vi "ACT_Loop.vi"() -> ()   [LabVIEW 2023, in "Shooter FX_ACT.lvlib"]
uses:
  Shooter FX_ACT.lvlib
  RoboRIO Utilities/Global_STOP.vi
  ENUM_ACT_Action.ctl
  ENUM_ACT_State.ctl
  Global_CMD_ACT_Data In.vi
  Global_ACT_Data Out.vi
  Cluster_CMD_ACT_Data.ctl
  <vilib>/Rock Robotics/WPI/MotorControl/WPI_MotorControlType.ctl
  <vilib>/Rock Robotics/SystemInterfaces/DIO/FPGA_DIOPWMChannel.ctl
  <vilib>/Rock Robotics/WPI/PWM/WPI_PWMDeadband.ctl
  <vilib>/Rock Robotics/SystemInterfaces/DIO/FPGA_DIOChannel.ctl
  <vilib>/Rock Robotics/WPI/MotorControl/WPI_MotorControlDeviceRef.ctl
  Shared Code/TypeDefs/Cluser_CAN Data.ctl
  <vilib>/Rock Robotics/WPI/ThirdParty/Phoenix-LabVIEW/Motor Controller/Controls/CTRE_Phoenix_MotorControl_NeutralMode.ctl
  Shared Code/TypeDefs/Cluster_FWD  REV Values.ctl
  Shared Code/TypeDefs/Cluster_PID Gains.ctl
  Cluster_Config HW Values.ctl
  b5508d6c-c1cc-4273-80c5-2077d34e1483.vi
  5f725c2a-0ce1-4524-8967-e83b15fdce90.vi
  <vilib>/Rock Robotics/WPI/ThirdParty/Phoenix-LabVIEW/Motor Controller/Controls/CTRE_Phoenix_MotorControl_ControlMode.ctl
  Shared Code/TypeDefs/Cluster_FX CloseLoop Values.ctl
  Shared Code/TypeDefs/Cluster_FX Current Values.ctl
  Cluster_HW Output Values.ctl
  ENUM_CMD_Mode Select.ctl
  Shared Code/TypeDefs/Cluster_FX Sensor Values.ctl
  4f1f8321-3dc8-4b28-8619-20673fc77ec2.vi
  Cluster_SW Output Data.ctl
  Cluster_Config SW Values.ctl
  36677ea0-a1a5-47a3-bc56-4475cb7c281e.vi
  573e44c0-11f4-4bd9-ad56-904ec25dba75.vi
  e7494af9-f670-4352-9dfa-ae6ce50709ea.vi
  6201c2b1-dcd8-4430-86f1-9b4ee56c7753.vi
  Shared Code/TypeDefs/Cluser_FX Config_Current Limits.ctl
  Shared Code/TypeDefs/Cluster_FX SLOT PID Config.ctl
  <vilib>/Rock Robotics/WPI/ThirdParty/Phoenix-LabVIEW/Motor Controller/Controls/CTRE_Phoenix_MotorControl_TalonFXInvertType.ctl
  Shared Code/TypeDefs/Cluster_Config FX Motor Output.ctl
  Shared Code/TypeDefs/Cluster_FX Voltage Values.ctl
  2024 Intake/Global_CMD_ACT_Data In.vi
  2024 Intake/Intake_ACT.lvlib
  2024 Intake/ENUM_Shooter_Mode.ctl
  2024 Intake/Cluster_CMD_ACT_Data.ctl
panel:
  in  "Enable 1":bool
  out "STATE":T1
  in  "CMD Override":T2(tab)
  in  "Percent Out":dbl(slide) scale=-1.0..1.0
  in  "Position Counts":dbl
  in  "Velocity Value":dbl
  out "Current Time":timestamp
  in  "SW Config":T3={"Ver"=0, "Shooting Speed (RPM)"=1000.0}
  out "SW Output":T4
  out "Sensor Read time":dbl format="%.3g"
  out "HW Sensors":T5
  in  "Read Saved Config":bool
  in  "Update Config":bool
  in  "HW Config":T10 {"CL"."Gains"."F" format="%#.8f"; "CL"."Gains"."D" format="%#.8f"; "CL"."Gains"."I" format="%#.8f"; "CL"."Gains"."P" format="%#.8f"; "Output"."Min"."REV" format="%.2f"; "Output"."Min"."FWD" format="%.2f"; "Output"."Max"."REV" format="%.2f"; "Output"."Max"."FWD" format="%.2f"}
  out "CMD":T19
  out "Cycle Time (S)":dbl format="%.3g"
  # "Teleop - Auto"
  # "Shoot at Target Speed"
  # "STOP"
  # "Tune Output\nto 1023 Max"
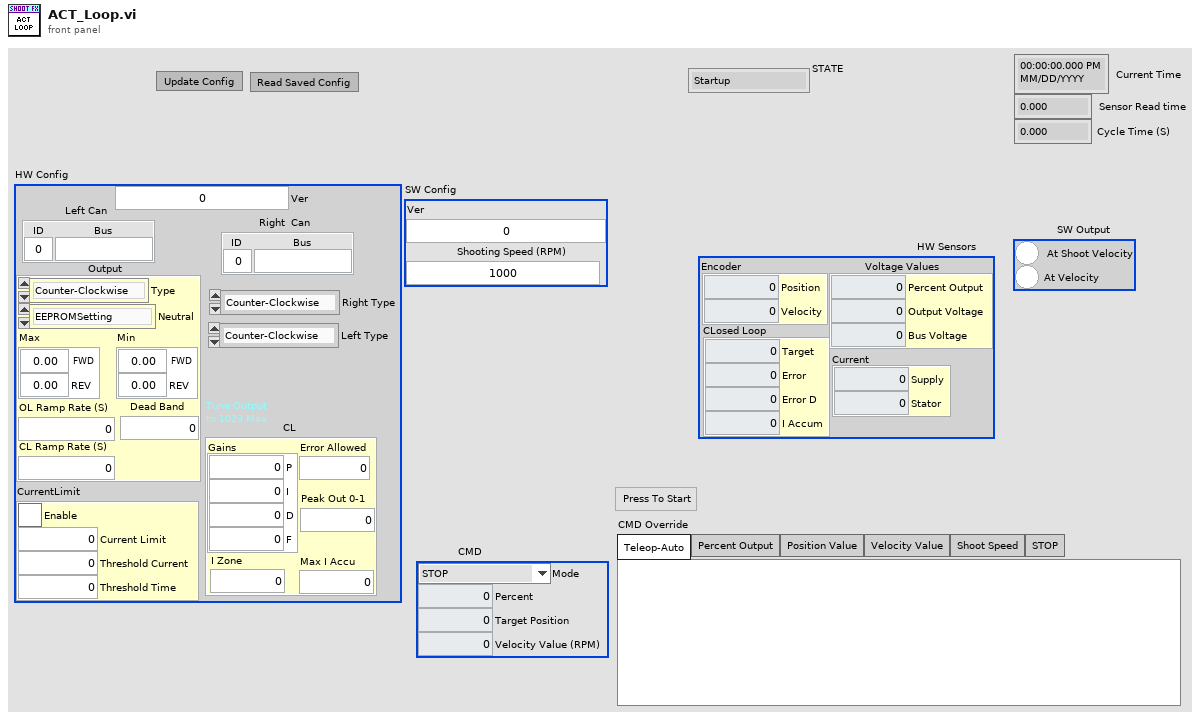
[diagram p1: front panel]
types:
  T1 = typedef "Shooter FX_ACT.lvlib/ENUM_ACT_State.ctl" = enum16{"Startup", "Configuring", "Stopping", "Moving Percent Out", "Moving to Position", "Shutdown", "Moving Velocity", "Moving to Shoot Vel", "Shooting"}
  T2 = enum32{"Teleop-Auto", "Percent Output", "Position Value", "Velocity Value", "Shoot Speed", "STOP"}
  T3 = typedef "Shooter FX_ACT.lvlib/Cluster_Config SW Values.ctl" = cluster{"Ver":u64, "Shooting Speed (RPM)":dbl}
  T4 = typedef "Shooter FX_ACT.lvlib/Cluster_SW Output Data.ctl" = cluster{"At Shoot Velocity":bool, "At Velocity":bool}
  T5 = typedef "Shooter FX_ACT.lvlib/Cluster_HW Output Values.ctl" = cluster{"Encoder":T6, "Current":T7, "CLosed Loop":T8, "Voltage Values":T9}
  T6 = typedef "Cluster_FX Sensor Values.ctl" = cluster{"Position":i32, "Velocity":i32}
  T7 = typedef "Cluster_FX Current Values.ctl" = cluster{"Supply":dbl, "Stator":dbl}
  T8 = typedef "Cluster_FX CloseLoop Values.ctl" = cluster{"Target":dbl, "Error":i32, "Error D":dbl, "I Accum":dbl}
  T9 = typedef "Cluster_FX Voltage Values.ctl" = cluster{"Percent Output":dbl, "Output Voltage":dbl, "Bus Voltage":dbl}
  T10 = typedef "Shooter FX_ACT.lvlib/Cluster_Config HW Values.ctl" = cluster{"Ver":u64, "Right  Can":T11, "Output":T12, "CL":T16, "CurrentLimit":T18, "Left Can":T11, "Right Type":T13, "Left Type":T13}
  T11 = typedef "Cluser_CAN Data.ctl" = cluster{"ID":u8, "Bus":string}
  T12 = typedef "Cluster_Config FX Motor Output.ctl" = cluster{"Type":T13, "Neutral":T14, "Max":T15, "Min":T15, "OL Ramp Rate (S)":dbl, "Dead Band":dbl, "CL Ramp Rate (S)":dbl}
  T13 = typedef "CTRE_Phoenix_MotorControl_TalonFXInvertType.ctl" = enum16{"Counter-Clockwise", "Clockwise"}
  T14 = typedef "CTRE_Phoenix_MotorControl_NeutralMode.ctl" = enum8{"EEPROMSetting", "Override to Coast", "Override to Brake"}
  T15 = typedef "Cluster_FWD  REV Values.ctl" = cluster{"FWD":dbl, "REV":dbl}
  T16 = typedef "Cluster_FX SLOT PID Config.ctl" = cluster{"Gains":T17, "Error Allowed":dbl, "I Zone":dbl, "Peak Out 0-1":dbl, "Max I Accu":dbl}
  T17 = typedef "Cluster_PID Gains.ctl" = cluster{"P":dbl, "I":dbl, "D":dbl, "F":dbl}
  T18 = typedef "Cluser_FX Config_Current Limits.ctl" = cluster{"Enable":bool, "Current Limit":dbl, "Threshold Current":dbl, "Threshold Time":dbl}
  T19 = typedef "Shooter FX_ACT.lvlib/Cluster_CMD_ACT_Data.ctl" = cluster{"Mode":T20, "Percent":dbl, "Target Position":dbl, "Velocity Value (RPM)":dbl}
  T20 = typedef "Shooter FX_ACT.lvlib/ENUM_CMD_Mode Select.ctl" = enum16{"STOP", "PercentOut", "Positon Value", "Velocity Value", "Shoot Speed", "Auto Shoot"}
  T21 = typedef "WPI_MotorControlDeviceRef.ctl" = cluster{"DeviceStatus":errorcluster, "Type":T22, "PWM":cluster{"PWM Channel":T23, "DeadBand":T24}, "CAN":cluster{"Device Number":u8, "SetOutput VI Ref":variant, "GetOutput VI Ref":variant, "Enable VI Ref":variant, "Disable VI Ref":variant, "Data":variant}, "Invert":bool, "DIO PWM":cluster{"PWM \"Enable\" Channel":T23, "DIOChannel":T25, "PWM Rate":dbl}}
  T22 = typedef "WPI_MotorControlType.ctl" = enum16{"PWM", "CAN", "DIO PWM"}
  T23 = typedef "FPGA_DIOPWMChannel.ctl" = enum8{"PWM 0", "PWM 1", "PWM 2", "PWM 3", "PWM 4", "PWM 5", "PWM 6", "PWM 7", "PWM 8", "PWM 9", "PWM MXP 0", "PWM MXP 1", "PWM MXP 2", "PWM MXP 3", "PWM MXP 4", "PWM MXP 5", "PWM MXP 6", "PWM MXP 7", "PWM MXP 8", "PWM MXP 9", "Invalid"}
  T24 = typedef "WPI_PWMDeadband.ctl" = cluster{"Name":string, "maxPositivePwm":i32, "minPositivePwm":i32, "centerPwm":i32, "maxNegativePwm":i32, "minNegativePwm":i32, "angularRange":u16}
  T25 = typedef "FPGA_DIOChannel.ctl" = enum8{"DIO 0", "DIO 1", "DIO 2", "DIO 3", "DIO 4", "DIO 5", "DIO 6", "DIO 7", "DIO 8", "DIO 9", "DIO MXP 0", "DIO MXP 1", "DIO MXP 2", "DIO MXP 3", "DIO MXP 4", "DIO MXP 5", "DIO MXP 6", "DIO MXP 7", "DIO MXP 8", "DIO MXP 9", "DIO MXP 10", "DIO MXP 11", "DIO MXP 12", "DIO MXP 13", "DIO MXP 14", "DIO MXP 15", "SPI Port CS1", "SPI Port CS2", "SPI Port CS3", "SPI Port MISO", "SPI Port MOSI", "Invalid"}
  T26 = typedef "Intake_ACT.lvlib/Cluster_CMD_ACT_Data.ctl" = cluster{"Mode":T27, "Speed Value":dbl}
  T27 = typedef "Intake_ACT.lvlib/ENUM_Shooter_Mode.ctl" = enum16{"Stop", "Speed Percent", "Speed RPM"}
  T28 = typedef "CTRE_Phoenix_MotorControl_ControlMode.ctl" = u16
  T29 = cluster{"Team Files Folder":path, "Left Motor":T21, "Right Motor Ref":T21, "State":T1, "Previous State":T1, "Current Time":timestamp, "Previous Time":timestamp, "Start Time":timestamp, "Target Time (ms)":u32, "Cycle Time(S)":dbl, "Update Display":bool, "ACT Input":T19, "HW Config":T10, "SW Config":T3, "Max # Of Config Tries":i32, "HW Out":T5, "SW Out":T4, "CAN Timeout":u32, "FX Mode":T28, "FX Set Value":dbl, "CMDIntake":T26}
  T30 = typedef "Shooter FX_ACT.lvlib/ENUM_ACT_Action.ctl" = enum16{"No Action", "Reset Time", "Reset All", "Config HW File Read", "Config HW File Save", "Config SW File Read", "Config SW File Save", "Config From FP", "Config HW Get", "Config HW Set", "Open HW Only", "Control FX Stop", "Control FX Set Percent Out", "Control FX Set Pos Value", "Control FX Set Velocity Value", "Control FX Set STOP", "Encoder Set to Zero", "Set Shooter Velocity"}
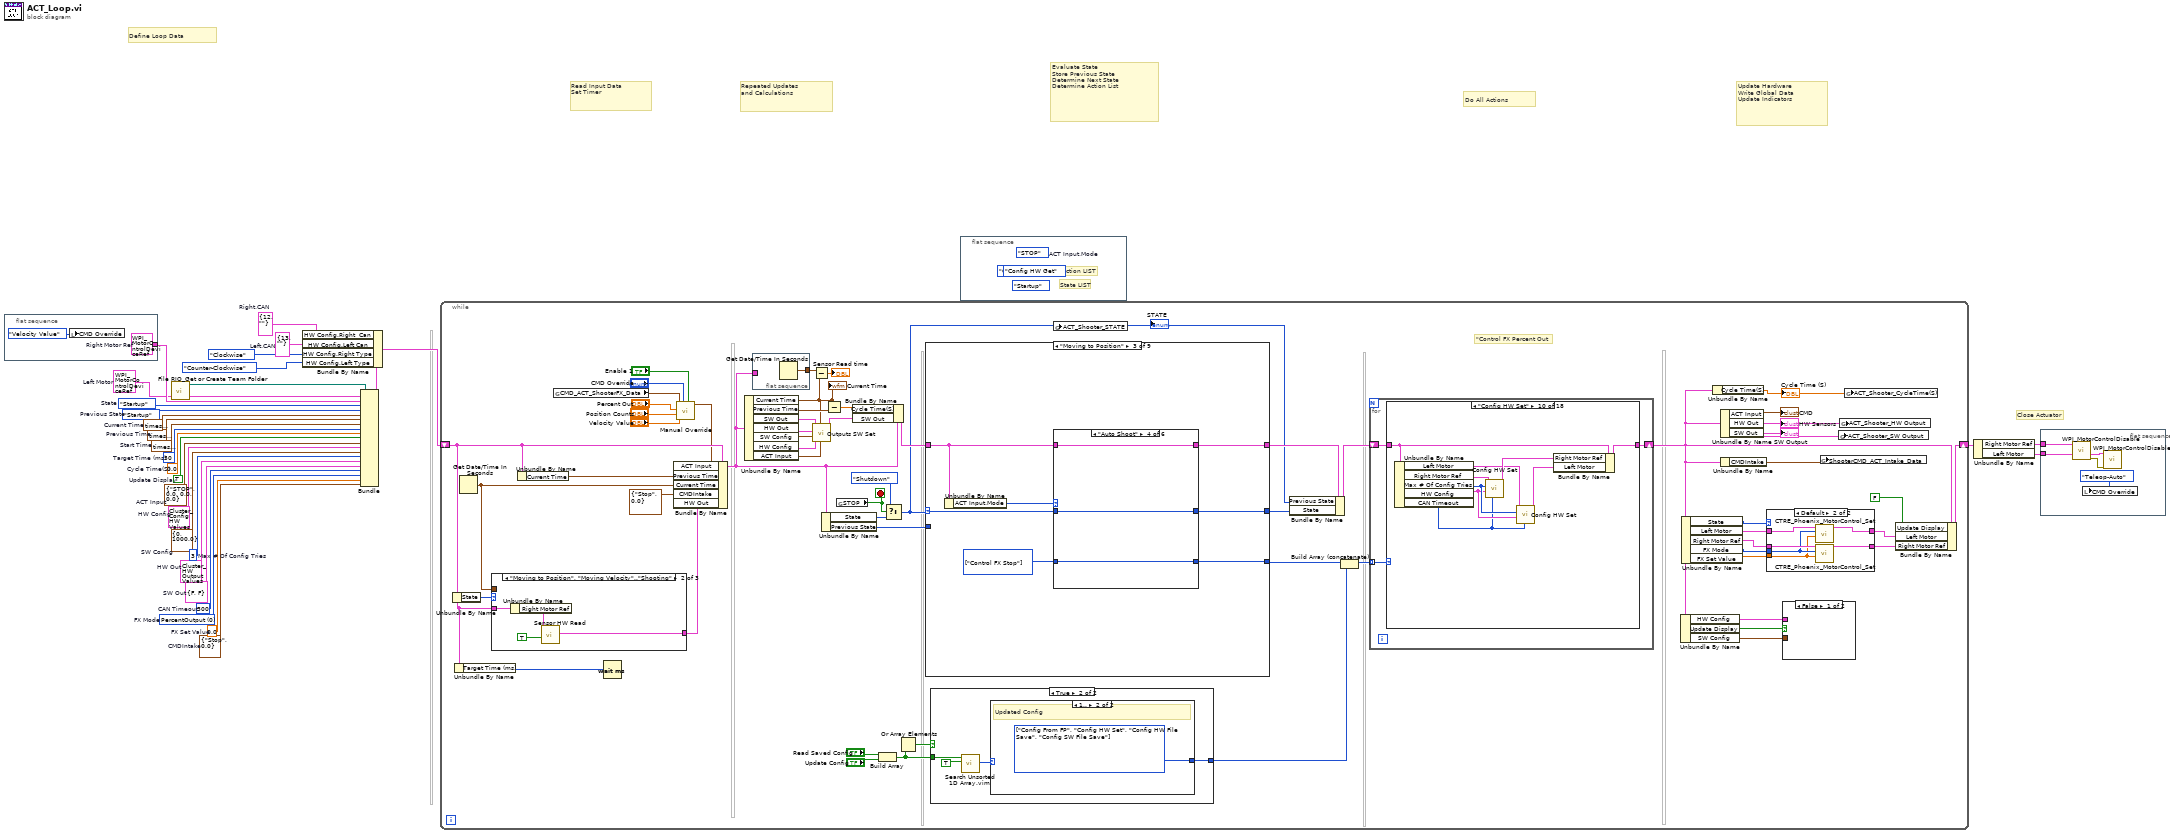
[diagram p0: block diagram]
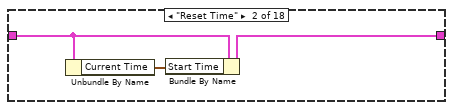
[diagram p3: hidden frame]
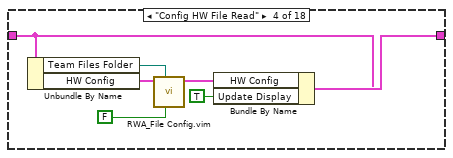
[diagram p5: hidden frame]
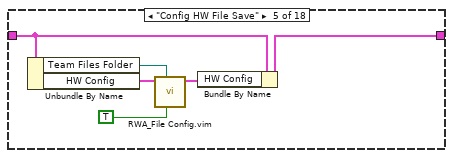
[diagram p6: hidden frame]
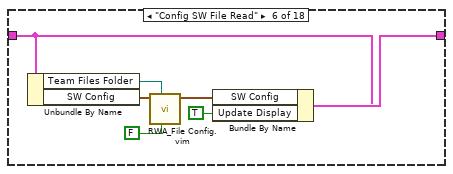
[diagram p7: hidden frame]
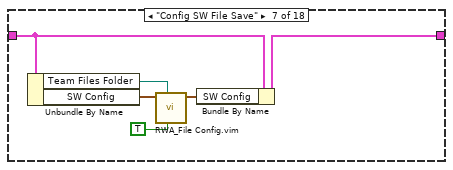
[diagram p8: hidden frame]
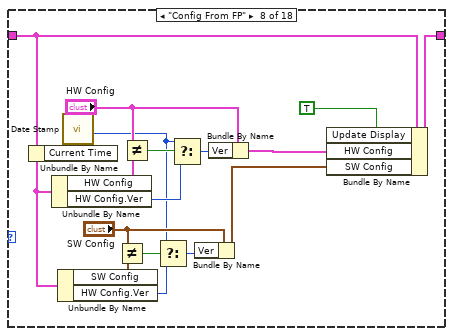
[diagram p9: hidden frame]
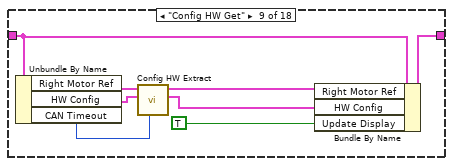
[diagram p10: hidden frame]
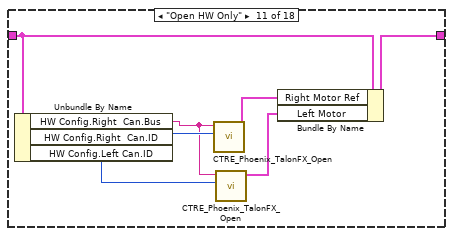
[diagram p11: hidden frame]
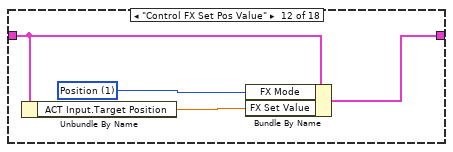
[diagram p12: hidden frame]
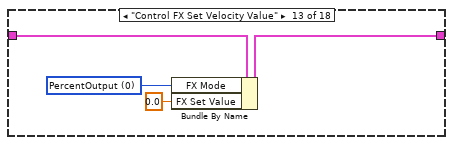
[diagram p13: hidden frame]
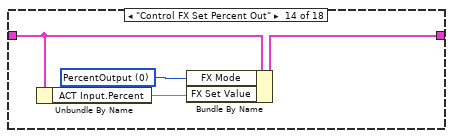
[diagram p14: hidden frame]
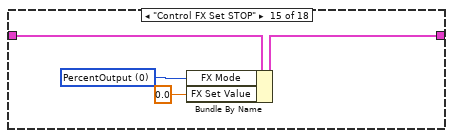
[diagram p15: hidden frame]
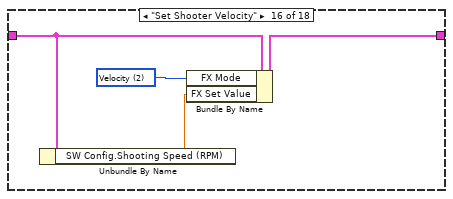
[diagram p16: hidden frame]
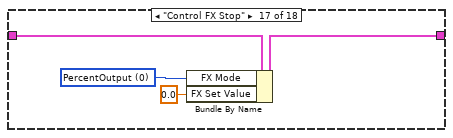
[diagram p17: hidden frame]
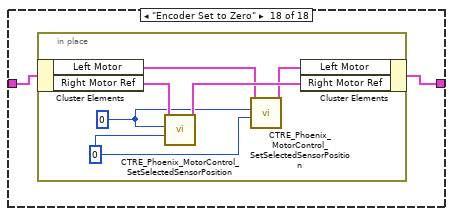
[diagram p18: hidden frame]
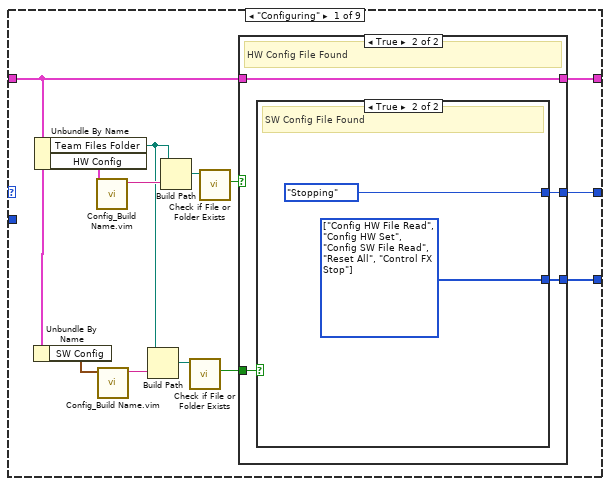
[diagram p19: hidden frame]
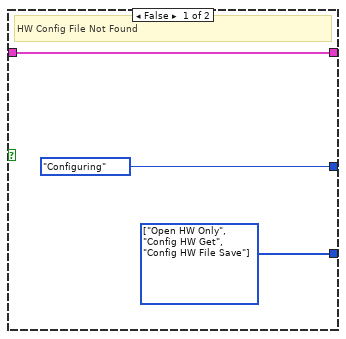
[diagram p20: hidden frame]
diagram:
  w3 = T11 {"ID"=13, "Bus"=""}  # Left.CAN
  w5 = T21 {"DeviceStatus"={"status"=FALSE, "code"=0, "source"=""}, "Type"=enum."PWM", "PWM"={"PWM Channel"=enum."PWM 1", "DeadBand"={"Name"="", "maxPositivePwm"=0, "minPositivePwm"=0, "centerPwm"=0, "maxNegativePwm"=0, "minNegativePwm"=0, "angularRange"=0}}, "CAN"={"Device Number"=0, "SetOutput VI Ref"=variant(enum8{"Percent VBus", "Current", "Speed", "Position", "Voltage"} enum."Percent VBus"), "GetOutput VI Ref"=variant(refnum<k1> refnum), "Enable VI Ref"=variant(dbl 12.0), "Disable VI Ref"=variant(enum8{"Percent VBus", "Speed", "Position", "Slave", "Unchanged / Invalid", "Voltage Compensation", "Current", "Motion Profile"} enum."Percent VBus"), "Data"=variant}, "Invert"=FALSE, "DIO PWM"={"PWM \"Enable\" Channel"=enum."Invalid", "DIOChannel"=enum."Invalid", "PWM Rate"=0.0}}  # Left Motor
  w6 = T26 {"Mode"=enum."Stop", "Speed Value"=0.0}  # CMDIntake
  w7 = T3 {"Ver"=0, "Shooting Speed (RPM)"=1000.0}  # SW Config
  w16 = T10 {"Ver"=0, "Right  Can"={"ID"=0, "Bus"=""}, "Output"={"Type"=enum."Counter-Clockwise", "Neutral"=enum."EEPROMSetting", "Max"={"FWD"=0.0, "REV"=0.0}, "Min"={"FWD"=0.0, "REV"=0.0}, "OL Ramp Rate (S)"=0.0, "Dead Band"=0.0, "CL Ramp Rate (S)"=0.0}, "CL"={"Gains"={"P"=0.0, "I"=0.0, "D"=0.0, "F"=0.0}, "Error Allowed"=0.0, "I Zone"=0.0, "Peak Out 0-1"=0.0, "Max I Accu"=0.0}, "CurrentLimit"={"Enable"=FALSE, "Current Limit"=0.0, "Threshold Current"=0.0, "Threshold Time"=0.0}, "Left Can"={"ID"=0, "Bus"=""}, "Right Type"=enum."Counter-Clockwise", "Left Type"=enum."Counter-Clockwise"}  # HW Config
  w14 = T4 {"At Shoot Velocity"=FALSE, "At Velocity"=FALSE}  # SW Out
  w15 = T5 {"Encoder"={"Position"=0, "Velocity"=0}, "Current"={"Supply"=0.0, "Stator"=0.0}, "CLosed Loop"={"Target"=0.0, "Error"=0, "Error D"=0.0, "I Accum"=0.0}, "Voltage Values"={"Percent Output"=0.0, "Output Voltage"=0.0, "Bus Voltage"=0.0}}  # HW Out
  w10 = 0.0  # FX Set Value
  w11 = T28 0 items=["PercentOutput"=0, "Position"=1, "Velocity"=2, "Current"=3, "Follower"=5, "MotionProfile"=6, "MotionMagic"=7, "MotionProfileArc"=10, "Disabled"=15]  # FX Mode
  w9 = u32 300  # CAN Timeout
  w8 = 3  # Max # Of Config Tries
  w18 = TRUE  # Update Display
  w19 = T11 {"ID"=12, "Bus"=""}  # Right.CAN
  w24 = 0.0  # Cycle Time(S)
  w25 = ENUM_ACT_State."Startup"  # Previous State
  w26 = timestamp(0 s since 1904-01-01)  # Previous Time
  w27 = u32 50  # Target Time (ms)
  w13 = T19 {"Mode"=enum."STOP", "Percent"=0.0, "Target Position"=0.0, "Velocity Value (RPM)"=0.0}  # ACT Input
  w28 = timestamp(0 s since 1904-01-01)  # Start Time
  w29 = timestamp(0 s since 1904-01-01)  # Current Time
  w30 = ENUM_ACT_State."Startup"  # State
  # "Close Actuator"
  # "Define Loop Data"
  # "Repeated Updates\nand Calculations"
  # "Read Input Data\nSet Timer"
  # "Evaluate State\nStore Previous State\nDetermine Next State\nDetermine Action List"
  # "Do All Actions"
  # "Update Hardware\nWrite Global Data\nUpdate Indicators"
  n1 = flat-sequence {
    tunnel: [w32] -> w20
    frame #0 {
      w32 = T21 {"DeviceStatus"={"status"=FALSE, "code"=0, "source"=""}, "Type"=enum."PWM", "PWM"={"PWM Channel"=enum."PWM 1", "DeadBand"={"Name"="", "maxPositivePwm"=0, "minPositivePwm"=0, "centerPwm"=0, "maxNegativePwm"=0, "minNegativePwm"=0, "angularRange"=0}}, "CAN"={"Device Number"=0, "SetOutput VI Ref"=variant(enum8{"Percent VBus", "Current", "Speed", "Position", "Voltage"} enum."Percent VBus"), "GetOutput VI Ref"=variant(refnum<k1> refnum), "Enable VI Ref"=variant(dbl 12.0), "Disable VI Ref"=variant(enum8{"Percent VBus", "Speed", "Position", "Slave", "Unchanged / Invalid", "Voltage Compensation", "Current", "Motion Profile"} enum."Percent VBus"), "Data"=variant}, "Invert"=FALSE, "DIO PWM"={"PWM \"Enable\" Channel"=enum."Invalid", "DIOChannel"=enum."Invalid", "PWM Rate"=0.0}}  # Right Motor Ref
      n2 = local write "CMD Override"(T2."Velocity Value" ("CMD Override")) -> ()
    }
  }
  n3 = call "File RIO_Get or Create Team Folder.vi"() -> ("Team Files Folder"=w12:path)  [unwired: 10 in, 1 out]
  n4 = Bundle("Team Files Folder"=w12, "Left Motor"=w5, "Right Motor Ref"=w20, "State"=w30, "Previous State"=w25, "Current Time"=w29, "Previous Time"=w26, "Start Time"=w28, "Target Time (ms)"=w27, "Cycle Time(S)"=w24, "Update Display"=w18, "ACT Input"=w13, "HW Config"=w16, "SW Config"=w7, "Max # Of Config Tries"=w8, "HW Out"=w15, "SW Out"=w14, "CAN Timeout"=w9, "FX Mode"=w11, "FX Set Value"=w10, "CMDIntake"=w6) -> (w22:T29)  [unwired: 1 in]
  n5 = Bundle By Name(cluster=w22, "HW Config.Right  Can"=w19, "HW Config.Left Can"=w3, "HW Config.Right Type"=CTRE_Phoenix_MotorControl_TalonFXInvertType."Clockwise", "HW Config.Left Type"=CTRE_Phoenix_MotorControl_TalonFXInvertType."Counter-Clockwise") -> (w21:T29)
  n6 = while {
    shift-right: [w76] -> w23
    shift-left: w21 -> [w47]
    stop <- w89 stop-if-true
    # "\"Control FX Percent Out"
    n7 = Unbundle By Name(w47) -> ("State"=w67:T1)
    n8 = Unbundle By Name(w47) -> ("Target Time (ms)"=w86:u32)
    n9 = Get Date/Time In Seconds() -> (seconds since 1Jan1904=w63:timestamp)
    n10 = case shown="\"Moving to Position\", \"Moving Velocity\"..\"Shooting\"" w67 {
      tunnel: w47 -> [w401 w405 _]
      tunnel: w63 -> [_ _ _]
      tunnel: [w398 w402 _] -> w48
      frame "Stopping", "Moving Percent Out" {
        n11 = Unbundle By Name(w401) -> ("Right Motor Ref"=w400:T21)
        n12 = call "Sensor HW Read.vi"("CloseLoop"=FALSE ("Read Closed Loop"), "PhoenixMotorControlDevRef"=w400) -> ("Sensor Values Out"=w398:T5)  [unwired: 7 in, 2 out]
      }
      frame "Moving to Position", "Moving Velocity".."Shooting" {
        n13 = Unbundle By Name(w405) -> ("Right Motor Ref"=w404:T21)
        n14 = call "Sensor HW Read.vi"("CloseLoop"=TRUE ("Read Closed Loop"), "PhoenixMotorControlDevRef"=w404) -> ("Sensor Values Out"=w402:T5)  [unwired: 7 in, 2 out]
      }
      frame "Startup", "Configuring", "Shutdown" {
      }
    }
    n15 = Unbundle By Name(w47) -> ("Current Time"=w85:timestamp)
    n16 = global read "Global_CMD_ACT_Data In.vi" "CMD_ACT_ShooterFX_Data"() -> (w44:T19)
    n17 = Wait (ms)(milliseconds to wait=w86) -> ()  [unwired: 1 out]
    n18 = call "Manual Override.vi"("Enable"="Enable 1", "CMD Override"="CMD Override", "Velocity Data"="Velocity Value", "Position Data"="Position Counts", "Percent Out Data"="Percent Out", "Auto CMD"=w44) -> ("OverRide Command Out"=w46:T19)  [unwired: 5 in]
    n19 = Bundle By Name(cluster=w47, "ACT Input"=w46, "Previous Time"=w85, "Current Time"=w63, "CMDIntake"=T26 {"Mode"=enum."Stop", "Speed Value"=0.0}, "HW Out"=w48) -> (w49:T29)
    n20 = Unbundle By Name(w49) -> ("Current Time"=w53:timestamp, "Previous Time"=w83:timestamp, "SW Out"=w56:T4, "HW Out"=w54:T5, "SW Config"=w52:T3, "HW Config"=w51:T10, "ACT Input"=w41:T19)
    "Current Time" <- w53
    n21 = flat-sequence {
      tunnel: [w93] -> w65
      tunnel: w49 -> [_]
      frame #0 {
        n22 = Get Date/Time In Seconds() -> (seconds since 1Jan1904=w93:timestamp)
      }
    }
    n23 = Subtract(x=w65, y=w53) -> (x-y=→"Sensor Read time":dbl)
    n24 = call "Outputs SW Set.vi"("CMD_ACT_Tempplate Data"=w41, "Current Time"=w53, "HW Config"=w51, "SW Config"=w52, "Sensor Values"=w54, "SW Output"=w56) -> ("SW Output Out"=w55:T4)  [unwired: 5 in]
    n25 = Unbundle By Name(w49) -> ("State"=w87:T1, "Previous State"=w84:T1)
    n26 = Subtract(x=w53, y=w83) -> (x-y=w81:dbl)
    n27 = global read "Global_STOP.vi" "STOP"() -> (w89:bool)
    n28 = Bundle By Name(cluster=w49, "Cycle Time(S)"=w81, "SW Out"=w55) -> (w82:T29)
    n29 = Build Array("Read Saved Config", "Update Config") -> (w59:bool[])
    n30 = Select(t=ENUM_ACT_State."Shutdown" ("State"), s=w89, f=w87) -> (s? t:f=w45:T1)
    "STATE" <- w45
    n31 = Or Array Elements(Boolean array=w59) -> (logical OR=w60:bool)
    n32 = case shown="\"Moving to Position\"" w45 {
      selector: w45 -> [_ w227 w252 w277 w302 w327 _ _ _]
      tunnel: w82 -> [w206 w228 w253 w278 w303 w328 w360 w363 w368]
      tunnel: [w209 w229 w254 w279 w304 w329 w360 w363 w367] -> w91
      tunnel: [w208 w231 w256 w281 w306 w331 ENUM_ACT_State."Shutdown" ("State") ENUM_ACT_State."Configuring" ("State") w366] -> w90
      tunnel: [w207 w226 w250 w275 w300 w325 w358 w362 w364] -> w80
      tunnel: w84 -> [_ _ _ _ _ _ _ _ _]
      frame "Configuring" {
        n33 = Unbundle By Name(w206) -> ("SW Config"=w204:T3)
        n34 = Unbundle By Name(w206) -> ("Team Files Folder"=w203:path, "HW Config"=w211:T10)
        n35 = call "Config_Build Name.vim"("Config First Name"=w211) -> ("Cfg file"=w213:string)  [unwired: 9 in, 1 out]
        n36 = call "Config_Build Name.vim"("Config First Name"=w204) -> ("Cfg file"=w205:string)  [unwired: 9 in, 1 out]
        n37 = Build Path(base path=w203, name or relative path=w205) -> (appended path=w202:path)
        n38 = Build Path(base path=w203, name or relative path=w213) -> (appended path=w212:path)
        n39 = call <vilib>:"Check if File or Folder Exists.vi"("path"=w202) -> ("file or folder exists?"=w201:bool)  [unwired: 8 in, 2 out]
        n40 = call <vilib>:"Check if File or Folder Exists.vi"("path"=w212) -> ("file or folder exists?"=w210:bool)  [unwired: 8 in, 2 out]
        n41 = case shown="True" w210 {
          tunnel: w206 -> [w216 w220]
          tunnel: [w216 w220] -> w209
          tunnel: [ENUM_ACT_State."Configuring" ("State") w219] -> w208
          tunnel: [w214 w218] -> w207
          tunnel: w201 -> [_ w217]
          frame False {
            w214 = T30[] [enum."Open HW Only", enum."Config HW Get", enum."Config HW File Save"] items=["No Action", "Reset Time", "Reset All", "Config HW File Read", "Config HW File Save", "Config SW File Read", "Config SW File Save", "Config From FP", "Config HW Get", "Config HW Set", "Open HW Only", "Control FX Stop", "Control FX Set Percent Out", "Control FX Set Pos Value", "Control FX Set Velocity Value", "Control FX Set STOP", "Encoder Set to Zero", "Set Shooter Velocity"] ("Actions")
            # "HW Config File Not Found"
          }
          frame True {
            # "HW Config File Found"
            n42 = case shown="True" w217 {
              tunnel: [ENUM_ACT_State."Configuring" ("State") ENUM_ACT_State."Stopping" ("State")] -> w219
              tunnel: [w221 w223] -> w218
              frame False {
                w221 = T30[] [enum."Config SW File Save"] items=["No Action", "Reset Time", "Reset All", "Config HW File Read", "Config HW File Save", "Config SW File Read", "Config SW File Save", "Config From FP", "Config HW Get", "Config HW Set", "Open HW Only", "Control FX Stop", "Control FX Set Percent Out", "Control FX Set Pos Value", "Control FX Set Velocity Value", "Control FX Set STOP", "Encoder Set to Zero", "Set Shooter Velocity"] ("Actions")
                # "SW Config File NOT Found"
              }
              frame True {
                w223 = T30[] [enum."Config HW File Read", enum."Config HW Set", enum."Config SW File Read", enum."Reset All", enum."Control FX Stop"] items=["No Action", "Reset Time", "Reset All", "Config HW File Read", "Config HW File Save", "Config SW File Read", "Config SW File Save", "Config From FP", "Config HW Get", "Config HW Set", "Open HW Only", "Control FX Stop", "Control FX Set Percent Out", "Control FX Set Pos Value", "Control FX Set Velocity Value", "Control FX Set STOP", "Encoder Set to Zero", "Set Shooter Velocity"] ("Actions")
                # "SW Config File Found"
              }
            }
          }
        }
      }
      frame "Moving Percent Out" {
        w225 = T30[] [enum."Control FX Stop"] items=["No Action", "Reset Time", "Reset All", "Config HW File Read", "Config HW File Save", "Config SW File Read", "Config SW File Save", "Config From FP", "Config HW Get", "Config HW Set", "Open HW Only", "Control FX Stop", "Control FX Set Percent Out", "Control FX Set Pos Value", "Control FX Set Velocity Value", "Control FX Set STOP", "Encoder Set to Zero", "Set Shooter Velocity"] ("Actions")
        n43 = Unbundle By Name(w228) -> ("ACT Input.Mode"=w230:T20)
        n44 = case shown="\"Auto Shoot\"" w230 {
          tunnel: [ENUM_ACT_State."Stopping" ("State") ENUM_ACT_State."Moving to Position" ("State") ENUM_ACT_State."Moving Velocity" ("State") ENUM_ACT_State."Moving to Shoot Vel" ("State") ENUM_ACT_State."Shooting" ("State") w248] -> w231
          tunnel: w228 -> [w234 w237 w240 w243 w246 w249]
          tunnel: [w234 w237 w240 w243 w246 w249] -> w229
          tunnel: w227 -> [_ _ _ _ _ w248]
          tunnel: [w232 w235 w238 w241 w244 w247] -> w226
          tunnel: w225 -> [w232 w235 w238 w241 w244 _]
          frame "STOP" {
          }
          frame "Positon Value" {
          }
          frame "Velocity Value" {
          }
          frame "Shoot Speed" {
          }
          frame "Auto Shoot" {
          }
          frame "PercentOut" {
            w247 = T30[] [enum."Control FX Set Percent Out"] items=["No Action", "Reset Time", "Reset All", "Config HW File Read", "Config HW File Save", "Config SW File Read", "Config SW File Save", "Config From FP", "Config HW Get", "Config HW Set", "Open HW Only", "Control FX Stop", "Control FX Set Percent Out", "Control FX Set Pos Value", "Control FX Set Velocity Value", "Control FX Set STOP", "Encoder Set to Zero", "Set Shooter Velocity"] ("Actions")
          }
        }
      }
      frame "Moving to Position" {
        w251 = T30[] [enum."Control FX Stop"] items=["No Action", "Reset Time", "Reset All", "Config HW File Read", "Config HW File Save", "Config SW File Read", "Config SW File Save", "Config From FP", "Config HW Get", "Config HW Set", "Open HW Only", "Control FX Stop", "Control FX Set Percent Out", "Control FX Set Pos Value", "Control FX Set Velocity Value", "Control FX Set STOP", "Encoder Set to Zero", "Set Shooter Velocity"] ("Actions")
        n45 = Unbundle By Name(w253) -> ("ACT Input.Mode"=w255:T20)
        n46 = case shown="\"Auto Shoot\"" w255 {
          tunnel: [ENUM_ACT_State."Stopping" ("State") w260 w264 w267 w270 ENUM_ACT_State."Moving Percent Out" ("State")] -> w256
          tunnel: w253 -> [w259 w262 w265 w268 w269 w274]
          tunnel: [w259 w262 w265 w268 w269 w274] -> w254
          tunnel: w252 -> [_ w260 w264 w267 w270 _]
          tunnel: [w257 w261 w263 w266 w271 w272] -> w250
          tunnel: w251 -> [w257 _ w263 w266 _ w272]
          frame "STOP" {
          }
          frame "Positon Value" {
            w261 = T30[] [enum."Control FX Set Pos Value"] items=["No Action", "Reset Time", "Reset All", "Config HW File Read", "Config HW File Save", "Config SW File Read", "Config SW File Save", "Config From FP", "Config HW Get", "Config HW Set", "Open HW Only", "Control FX Stop", "Control FX Set Percent Out", "Control FX Set Pos Value", "Control FX Set Velocity Value", "Control FX Set STOP", "Encoder Set to Zero", "Set Shooter Velocity"] ("Actions")
          }
          frame "Shoot Speed" {
          }
          frame "Auto Shoot" {
          }
          frame "Velocity Value" {
            w271 = T30[] [enum."Control FX Set Velocity Value"] items=["No Action", "Reset Time", "Reset All", "Config HW File Read", "Config HW File Save", "Config SW File Read", "Config SW File Save", "Config From FP", "Config HW Get", "Config HW Set", "Open HW Only", "Control FX Stop", "Control FX Set Percent Out", "Control FX Set Pos Value", "Control FX Set Velocity Value", "Control FX Set STOP", "Encoder Set to Zero", "Set Shooter Velocity"] ("Actions")
          }
          frame "PercentOut" {
          }
        }
      }
      frame "Moving Velocity" {
        w276 = T30[] [enum."Control FX Stop"] items=["No Action", "Reset Time", "Reset All", "Config HW File Read", "Config HW File Save", "Config SW File Read", "Config SW File Save", "Config From FP", "Config HW Get", "Config HW Set", "Open HW Only", "Control FX Stop", "Control FX Set Percent Out", "Control FX Set Pos Value", "Control FX Set Velocity Value", "Control FX Set STOP", "Encoder Set to Zero", "Set Shooter Velocity"] ("Actions")
        n47 = Unbundle By Name(w278) -> ("ACT Input.Mode"=w280:T20)
        n48 = case shown="\"PercentOut\"" w280 {
          tunnel: [ENUM_ACT_State."Stopping" ("State") ENUM_ACT_State."Moving to Position" ("State") ENUM_ACT_State."Moving to Shoot Vel" ("State") ENUM_ACT_State."Shooting" ("State") w295 ENUM_ACT_State."Moving Percent Out" ("State")] -> w281
          tunnel: w278 -> [w284 w287 w290 w293 w294 w299]
          tunnel: [w284 w287 w290 w293 w294 w299] -> w279
          tunnel: w277 -> [_ _ _ _ w295 _]
          tunnel: [w282 w286 w288 w291 w296 w297] -> w275
          tunnel: w276 -> [w282 w286 w288 w291 _ w297]
          frame "STOP" {
          }
          frame "Positon Value" {
          }
          frame "Shoot Speed" {
          }
          frame "Auto Shoot" {
          }
          frame "Velocity Value" {
            w296 = T30[] [enum."Control FX Set Velocity Value"] items=["No Action", "Reset Time", "Reset All", "Config HW File Read", "Config HW File Save", "Config SW File Read", "Config SW File Save", "Config From FP", "Config HW Get", "Config HW Set", "Open HW Only", "Control FX Stop", "Control FX Set Percent Out", "Control FX Set Pos Value", "Control FX Set Velocity Value", "Control FX Set STOP", "Encoder Set to Zero", "Set Shooter Velocity"] ("Actions")
          }
          frame "PercentOut" {
          }
        }
      }
      frame "Moving to Shoot Vel" {
        w301 = T30[] [enum."Control FX Stop"] items=["No Action", "Reset Time", "Reset All", "Config HW File Read", "Config HW File Save", "Config SW File Read", "Config SW File Save", "Config From FP", "Config HW Get", "Config HW Set", "Open HW Only", "Control FX Stop", "Control FX Set Percent Out", "Control FX Set Pos Value", "Control FX Set Velocity Value", "Control FX Set STOP", "Encoder Set to Zero", "Set Shooter Velocity"] ("Actions")
        n49 = Unbundle By Name(w303) -> ("ACT Input.Mode"=w305:T20)
        n50 = case shown="\"PercentOut\"" w305 {
          tunnel: [ENUM_ACT_State."Stopping" ("State") ENUM_ACT_State."Moving to Position" ("State") ENUM_ACT_State."Moving to Shoot Vel" ("State") ENUM_ACT_State."Shooting" ("State") ENUM_ACT_State."Moving Velocity" ("State") ENUM_ACT_State."Moving Percent Out" ("State")] -> w306
          tunnel: w303 -> [w309 w312 w315 w318 w321 w324]
          tunnel: [w309 w312 w315 w318 w321 w324] -> w304
          tunnel: w302 -> [_ _ _ _ _ _]
          tunnel: [w307 w311 w313 w316 w319 w322] -> w300
          tunnel: w301 -> [w307 w311 _ w316 w319 w322]
          frame "STOP" {
          }
          frame "Positon Value" {
          }
          frame "Shoot Speed" {
            w313 = T30[] [enum."Set Shooter Velocity"] items=["No Action", "Reset Time", "Reset All", "Config HW File Read", "Config HW File Save", "Config SW File Read", "Config SW File Save", "Config From FP", "Config HW Get", "Config HW Set", "Open HW Only", "Control FX Stop", "Control FX Set Percent Out", "Control FX Set Pos Value", "Control FX Set Velocity Value", "Control FX Set STOP", "Encoder Set to Zero", "Set Shooter Velocity"] ("Actions")
          }
          frame "Auto Shoot" {
          }
          frame "Velocity Value" {
          }
          frame "PercentOut" {
          }
        }
      }
      frame "Shooting" {
        w326 = T30[] [enum."Control FX Stop"] items=["No Action", "Reset Time", "Reset All", "Config HW File Read", "Config HW File Save", "Config SW File Read", "Config SW File Save", "Config From FP", "Config HW Get", "Config HW Set", "Open HW Only", "Control FX Stop", "Control FX Set Percent Out", "Control FX Set Pos Value", "Control FX Set Velocity Value", "Control FX Set STOP", "Encoder Set to Zero", "Set Shooter Velocity"] ("Actions")
        n51 = Unbundle By Name(w328) -> ("ACT Input.Mode"=w330:T20)
        n52 = case shown="\"Auto Shoot\"" w330 {
          tunnel: [ENUM_ACT_State."Stopping" ("State") ENUM_ACT_State."Moving to Position" ("State") ENUM_ACT_State."Moving to Shoot Vel" ("State") ENUM_ACT_State."Shooting" ("State") ENUM_ACT_State."Moving to Shoot Vel" ("State") ENUM_ACT_State."Moving Percent Out" ("State")] -> w331
          tunnel: w328 -> [w334 w337 w340 w342 w354 w357]
          tunnel: [w334 w337 w340 w343 w354 w357] -> w329
          tunnel: w327 -> [_ _ _ _ _ _]
          tunnel: [w332 w336 w338 w344 w353 w355] -> w325
          tunnel: w326 -> [w332 w336 w338 _ w353 w355]
          frame "STOP" {
          }
          frame "Positon Value" {
          }
          frame "Shoot Speed" {
          }
          frame "Auto Shoot" {
            w344 = T30[] [enum."Set Shooter Velocity"] items=["No Action", "Reset Time", "Reset All", "Config HW File Read", "Config HW File Save", "Config SW File Read", "Config SW File Save", "Config From FP", "Config HW Get", "Config HW Set", "Open HW Only", "Control FX Stop", "Control FX Set Percent Out", "Control FX Set Pos Value", "Control FX Set Velocity Value", "Control FX Set STOP", "Encoder Set to Zero", "Set Shooter Velocity"] ("Actions")
            n53 = Unbundle By Name(w342) -> ("SW Out.At Shoot Velocity"=w341:bool)
            n54 = case shown="False" w341 {
              tunnel: [w348 w351] -> w343
              tunnel: w342 -> [w347 w350]
              frame True {
                n55 = Bundle By Name(cluster=w347, "CMDIntake"=T26 {"Mode"=enum."Speed Percent", "Speed Value"=0.7}) -> (w348:T29)
              }
              frame False {
                n56 = Bundle By Name(cluster=w350, "CMDIntake"=T26 {"Mode"=enum."Stop", "Speed Value"=0.0}) -> (w351:T29)
              }
            }
          }
          frame "Velocity Value" {
          }
          frame "PercentOut" {
          }
        }
      }
      frame "Shutdown" {
        w358 = T30[] [enum."Reset All"] items=["No Action", "Reset Time", "Reset All", "Config HW File Read", "Config HW File Save", "Config SW File Read", "Config SW File Save", "Config From FP", "Config HW Get", "Config HW Set", "Open HW Only", "Control FX Stop", "Control FX Set Percent Out", "Control FX Set Pos Value", "Control FX Set Velocity Value", "Control FX Set STOP", "Encoder Set to Zero", "Set Shooter Velocity"] ("Actions")
      }
      frame "Startup" {
        w362 = T30[] [enum."Reset Time"] items=["No Action", "Reset Time", "Reset All", "Config HW File Read", "Config HW File Save", "Config SW File Read", "Config SW File Save", "Config From FP", "Config HW Get", "Config HW Set", "Open HW Only", "Control FX Stop", "Control FX Set Percent Out", "Control FX Set Pos Value", "Control FX Set Velocity Value", "Control FX Set STOP", "Encoder Set to Zero", "Set Shooter Velocity"] ("Actions")
      }
      frame "Stopping" {
        (unwired) TRUE
        w365 = T30[] [enum."Control FX Stop"] items=["No Action", "Reset Time", "Reset All", "Config HW File Read", "Config HW File Save", "Config SW File Read", "Config SW File Save", "Config From FP", "Config HW Get", "Config HW Set", "Open HW Only", "Control FX Stop", "Control FX Set Percent Out", "Control FX Set Pos Value", "Control FX Set Velocity Value", "Control FX Set STOP", "Encoder Set to Zero", "Set Shooter Velocity"] ("Actions")
        n57 = Unbundle By Name(w368) -> ("ACT Input.Mode"=w369:T20)
        n58 = case shown="\"Shoot Speed\"" w369 {
          tunnel: w368 -> [w372 w375 w378 w381 w384 w387]
          tunnel: [w372 w375 w378 w381 w384 w387] -> w367
          tunnel: [ENUM_ACT_State."Stopping" ("State") ENUM_ACT_State."Moving Percent Out" ("State") ENUM_ACT_State."Moving to Shoot Vel" ("State") ENUM_ACT_State."Shooting" ("State") ENUM_ACT_State."Moving to Position" ("State") ENUM_ACT_State."Moving Velocity" ("State")] -> w366
          tunnel: [w370 w373 w376 w379 w382 w385] -> w364
          tunnel: w365 -> [w370 w373 w376 w379 w382 w385]
          frame "STOP" {
          }
          frame "PercentOut" {
          }
          frame "Shoot Speed" {
          }
          frame "Auto Shoot" {
          }
          frame "Positon Value" {
          }
          frame "Velocity Value" {
          }
        }
      }
    }
    n59 = case shown="True" w60 {
      tunnel: w59 -> [_ w408]
      tunnel: [_ w406] -> w58
      frame False {
      }
      frame True {
        n60 = call "Search Unsorted 1D Array.vim"("element"=TRUE, "unsorted 1D array"=w408) -> ("index of element"=w407:i32)  [unwired: 9 in]
        n61 = case shown="1.." w407 {
          tunnel: [w410 w411] -> w406
          frame ..0 {
            w410 = T30[] [enum."Config HW File Read", enum."Config HW Set", enum."Config SW File Read"] items=["No Action", "Reset Time", "Reset All", "Config HW File Read", "Config HW File Save", "Config SW File Read", "Config SW File Save", "Config From FP", "Config HW Get", "Config HW Set", "Open HW Only", "Control FX Stop", "Control FX Set Percent Out", "Control FX Set Pos Value", "Control FX Set Velocity Value", "Control FX Set STOP", "Encoder Set to Zero", "Set Shooter Velocity"] ("Actions")
            # "Read Config"
          }
          frame 1.. {
            w411 = T30[] [enum."Config From FP", enum."Config HW Set", enum."Config HW File Save", enum."Config SW File Save"] items=["No Action", "Reset Time", "Reset All", "Config HW File Read", "Config HW File Save", "Config SW File Read", "Config SW File Save", "Config From FP", "Config HW Get", "Config HW Set", "Open HW Only", "Control FX Stop", "Control FX Set Percent Out", "Control FX Set Pos Value", "Control FX Set Velocity Value", "Control FX Set STOP", "Encoder Set to Zero", "Set Shooter Velocity"] ("Actions")
            # "Updated Config"
          }
        }
      }
    }
    n62 = global write "Global_ACT_Data Out.vi" "ACT_Shooter_STATE"(w45) -> ()
    n63 = Bundle By Name(cluster=w91, "Previous State"=w45, "State"=w90) -> (w92:T29)
    n64 = Build Array (concatenate)(w80, w58) -> (w74:T30[])
    n65 = for {
      tunnel: w74 -> [w96] mode=indexing
      shift-right: [w95] -> w37
      shift-left: w92 -> [w94]
      n66 = case shown="\"Config HW Set\"" w96 {
        tunnel: w94 -> [w97 w100 w101 w107 w113 w120 w126 w134 w149 w159 w165 w170 w174 w178 w182 w186 w190 w194]
        tunnel: [w97 w99 w101 w108 w114 w121 w127 w144 w150 w160 w166 w172 w176 w180 w184 w188 w192 w193] -> w95
        frame "No Action" {
        }
        frame "Reset Time" {
          n67 = Unbundle By Name(w100) -> ("Current Time"=w98:timestamp)
          n68 = Bundle By Name(cluster=w100, "Start Time"=w98) -> (w99:T29)
        }
        frame "Reset All" {
        }
        frame "Config HW File Read" {
          n69 = Unbundle By Name(w107) -> ("Team Files Folder"=w105:path, "HW Config"=w102:T10)
          n70 = call "RWA_File Config.vim"("Read(f) Save(t)"=FALSE ("Read(f) Write(t)"), "Target Folder Folder"=w105, "Any Config"=w102) -> ("Any Config Out"=w106:T10)  [unwired: 4 in, 4 out]
          n71 = Bundle By Name(cluster=w107, "HW Config"=w106, "Update Display"=TRUE) -> (w108:T29)
        }
        frame "Config HW File Save" {
          n72 = Unbundle By Name(w113) -> ("Team Files Folder"=w111:path, "HW Config"=w109:T10)
          n73 = call "RWA_File Config.vim"("Read(f) Save(t)"=TRUE ("Read(f) Write(t)"), "Target Folder Folder"=w111, "Any Config"=w109) -> ("Any Config Out"=w112:T10)  [unwired: 4 in, 4 out]
          n74 = Bundle By Name(cluster=w113, "HW Config"=w112) -> (w114:T29)
        }
        frame "Config SW File Read" {
          n75 = Unbundle By Name(w120) -> ("Team Files Folder"=w117:path, "SW Config"=w119:T3)
          n76 = call "RWA_File Config.vim"("Read(f) Save(t)"=FALSE ("Read(f) Write(t)"), "Target Folder Folder"=w117, "Any Config"=w119) -> ("Any Config Out"=w118:T3)  [unwired: 4 in, 4 out]
          n77 = Bundle By Name(cluster=w120, "SW Config"=w118, "Update Display"=TRUE) -> (w121:T29)
        }
        frame "Config SW File Save" {
          n78 = Unbundle By Name(w126) -> ("Team Files Folder"=w123:path, "SW Config"=w125:T3)
          n79 = call "RWA_File Config.vim"("Read(f) Save(t)"=TRUE ("Read(f) Write(t)"), "Target Folder Folder"=w123, "Any Config"=w125) -> ("Any Config Out"=w124:T3)  [unwired: 4 in, 4 out]
          n80 = Bundle By Name(cluster=w126, "SW Config"=w124) -> (w127:T29)
        }
        frame "Config From FP" {
          n81 = Unbundle By Name(w134) -> ("Current Time"=w143:timestamp)
          n82 = Unbundle By Name(w134) -> ("HW Config"=w133:T10, "HW Config.Ver"=w130:u64)
          n83 = Unbundle By Name(w134) -> ("SW Config"=w136:T3, "HW Config.Ver"=w138:u64)
          n84 = call "Date Stamp.vi"("Time"=w143) -> ("U64 Out"=w129:u64)  [unwired: 5 in, 1 out]
          n85 = Not Equal?(x=w136, y="SW Config") -> (x != y?=w139:bool)
          n86 = Not Equal?(x="HW Config", y=w133) -> (x != y?=w131:bool)
          n87 = Select(t=w129, s=w139, f=w138) -> (s? t:f=w137:u64)
          n88 = Select(t=w129, s=w131, f=w130) -> (s? t:f=w128:u64)
          n89 = Bundle By Name(cluster="SW Config", "Ver"=w137) -> (w141:T3)
          n90 = Bundle By Name(cluster="HW Config", "Ver"=w128) -> (w142:T10)
          n91 = Bundle By Name(cluster=w134, "Update Display"=TRUE, "HW Config"=w142, "SW Config"=w141) -> (w144:T29)
        }
        frame "Config HW Get" {
          n92 = Unbundle By Name(w149) -> ("Right Motor Ref"=w152:T21, "HW Config"=w151:T10, "CAN Timeout"=w145:u32)
          n93 = call "Config HW Extract.vi"("Send Cmd Timout(ms)"=w145, "HW Config"=w151, "DevRef"=w152) -> ("HW Config Data Out"=w147:T10, "DevRef Out"=w148:T21)  [unwired: 6 in, 1 out]
          n94 = Bundle By Name(cluster=w149, "Right Motor Ref"=w148, "HW Config"=w147, "Update Display"=TRUE) -> (w150:T29)
        }
        frame "Config HW Set" {
          n95 = Unbundle By Name(w159) -> ("Left Motor"=w157:T21, "Right Motor Ref"=w161:T21, "Max # Of Config Tries"=w155:i32, "HW Config"=w154:T10, "CAN Timeout"=w153:u32)
          n96 = call "Config HW Set.vi"("Send Cmd Timout(ms)"=w153, "Wrist Config"=w154, "Max # Of Tries"=w155, "DevRef"=w161) -> ("DevRef Out Out"=w158:T21)  [unwired: 6 in, 1 out]
          n97 = call "Config HW Set.vi"("Send Cmd Timout(ms)"=w153, "Wrist Config"=w154, "Max # Of Tries"=w155, "DevRef"=w157) -> ("DevRef Out Out"=w156:T21)  [unwired: 6 in, 1 out]
          n98 = Bundle By Name(cluster=w159, "Right Motor Ref"=w158, "Left Motor"=w156) -> (w160:T29)
        }
        frame "Open HW Only" {
          n99 = Unbundle By Name(w165) -> ("HW Config.Right  Can.Bus"=w163:string, "HW Config.Right  Can.ID"=w168:u8, "HW Config.Left Can.ID"=w162:u8)
          n100 = call <vilib>:"CTRE_Phoenix_TalonFX_Open.vi"("Device Number"=w168, "CAN Bus"=w163) -> ("PhoenixMotorControlDevRef"=w167:T21)  [unwired: 8 in, 1 out]
          n101 = call <vilib>:"CTRE_Phoenix_TalonFX_Open.vi"("Device Number"=w162, "CAN Bus"=w163) -> ("PhoenixMotorControlDevRef"=w164:T21)  [unwired: 8 in, 1 out]
          n102 = Bundle By Name(cluster=w165, "Right Motor Ref"=w167, "Left Motor"=w164) -> (w166:T29)
        }
        frame "Control FX Set Pos Value" {
          w171 = T28 1 items=["PercentOutput"=0, "Position"=1, "Velocity"=2, "Current"=3, "Follower"=5, "MotionProfile"=6, "MotionMagic"=7, "MotionProfileArc"=10, "Disabled"=15] ("FX Mode")
          n103 = Unbundle By Name(w170) -> ("ACT Input.Target Position"=w169:dbl)
          n104 = Bundle By Name(cluster=w170, "FX Mode"=w171, "FX Set Value"=w169) -> (w172:T29)
        }
        frame "Control FX Set Velocity Value" {
          w175 = T28 0 items=["PercentOutput"=0, "Position"=1, "Velocity"=2, "Current"=3, "Follower"=5, "MotionProfile"=6, "MotionMagic"=7, "MotionProfileArc"=10, "Disabled"=15] ("FX Mode")
          n105 = Bundle By Name(cluster=w174, "FX Mode"=w175, "FX Set Value"=0.0) -> (w176:T29)
        }
        frame "Control FX Set Percent Out" {
          w179 = T28 0 items=["PercentOutput"=0, "Position"=1, "Velocity"=2, "Current"=3, "Follower"=5, "MotionProfile"=6, "MotionMagic"=7, "MotionProfileArc"=10, "Disabled"=15] ("FX Mode")
          n106 = Unbundle By Name(w178) -> ("ACT Input.Percent"=w177:dbl)
          n107 = Bundle By Name(cluster=w178, "FX Mode"=w179, "FX Set Value"=w177) -> (w180:T29)
        }
        frame "Control FX Set STOP" {
          w183 = T28 0 items=["PercentOutput"=0, "Position"=1, "Velocity"=2, "Current"=3, "Follower"=5, "MotionProfile"=6, "MotionMagic"=7, "MotionProfileArc"=10, "Disabled"=15] ("FX Mode")
          n108 = Bundle By Name(cluster=w182, "FX Mode"=w183, "FX Set Value"=0.0 ("HW Out.Set.Value")) -> (w184:T29)
        }
        frame "Set Shooter Velocity" {
          w187 = T28 2 items=["PercentOutput"=0, "Position"=1, "Velocity"=2, "Current"=3, "Follower"=5, "MotionProfile"=6, "MotionMagic"=7, "MotionProfileArc"=10, "Disabled"=15] ("FX Mode")
          n109 = Unbundle By Name(w186) -> ("SW Config.Shooting Speed (RPM)"=w185:dbl)
          n110 = Bundle By Name(cluster=w186, "FX Mode"=w187, "FX Set Value"=w185) -> (w188:T29)
        }
        frame "Control FX Stop" {
          w191 = T28 0 items=["PercentOutput"=0, "Position"=1, "Velocity"=2, "Current"=3, "Follower"=5, "MotionProfile"=6, "MotionMagic"=7, "MotionProfileArc"=10, "Disabled"=15] ("FX Mode")
          n111 = Bundle By Name(cluster=w190, "FX Mode"=w191, "FX Set Value"=0.0) -> (w192:T29)
        }
        frame "Encoder Set to Zero" {
          n112 = in-place {
            w195 = u32 0 ("pidLoopIdx")
            w196 = 0 ("New Sensor Position")
            n113 = in-place-cluster #1(w194) -> ("Left Motor"=w198:T21, "Right Motor Ref"=w200:T21)
            n114 = call <vilib>:"CTRE_Phoenix_MotorControl_SetSelectedSensorPosition.vi"("pidLoopIdx"=w195, "New Sensor Position"=w196, "PhoenixMotorControlDevRef"=w200) -> ("PhoenixMotorControlDevRef"=w199:T21)  [unwired: 7 in, 1 out]
            n115 = call <vilib>:"CTRE_Phoenix_MotorControl_SetSelectedSensorPosition.vi"("pidLoopIdx"=w195, "New Sensor Position"=w196, "PhoenixMotorControlDevRef"=w198) -> ("PhoenixMotorControlDevRef"=w197:T21)  [unwired: 7 in, 1 out]
            n116 = in-place-cluster #1("Left Motor"=w197, "Right Motor Ref"=w199) -> (w193:T29)
          }
        }
      }
    }
    n117 = Unbundle By Name(w37) -> ("HW Config"=w71:T10, "Update Display"=w72:bool, "SW Config"=w50:T3)
    n118 = Unbundle By Name(w37) -> ("State"=w68:T1, "Left Motor"=w34:T21, "Right Motor Ref"=w78:T21, "FX Mode"=w69:T28, "FX Set Value"=w70:dbl)
    n119 = Unbundle By Name(w37) -> ("Cycle Time(S)"=w75:dbl)
    "Cycle Time (S)" <- w75
    n120 = Unbundle By Name(w37) -> ("ACT Input"=→"CMD":T19, "HW Out"=w66:T5, "SW Out"=w57:T4)
    "HW Sensors" <- w66
    "SW Output" <- w57
    n121 = Unbundle By Name(w37) -> ("CMDIntake"=w36:T26)
    n122 = case shown="Default" w68 {
      tunnel: w78 -> [w389 w395]
      tunnel: [w389 w394] -> w77
      tunnel: w70 -> [_ w391]
      tunnel: w69 -> [_ w392]
      tunnel: w34 -> [w388 w393]
      tunnel: [w388 w390] -> w33
      frame "Startup", "Configuring" {
      }
      frame Default {
        n123 = call <vilib>:"CTRE_Phoenix_MotorControl_Set.vi"("Output"=w391, "Control Mode"=w392, "PhoenixMotorControlDevRef"=w393) -> ("PhoenixMotorControlDevRef"=w390:T21)  [unwired: 7 in, 1 out]
        n124 = call <vilib>:"CTRE_Phoenix_MotorControl_Set.vi"("Output"=w391, "Control Mode"=w392, "PhoenixMotorControlDevRef"=w395) -> ("PhoenixMotorControlDevRef"=w394:T21)  [unwired: 7 in, 1 out]
      }
    }
    n125 = case shown="False" w72 {
      tunnel: w71 -> [_ w397]
      tunnel: w50 -> [_ w396]
      frame False {
      }
      frame True {
        n126 = local write "SW Config"(w396) -> ()
        n127 = local write "HW Config"(w397) -> ()
      }
    }
    n128 = global write "Global_CMD_ACT_Data In.vi" "ShooterCMD_ACT_Intake_Data"(w36) -> ()
    n129 = global write "Global_ACT_Data Out.vi" "ACT_Shooter_SW Output"(w57) -> ()
    n130 = global write "Global_ACT_Data Out.vi" "ACT_Shooter_HW Output"(w66) -> ()
    n131 = global write "Global_ACT_Data Out.vi" "ACT_Shooter_CycleTime(S)"(w75) -> ()
    n132 = Bundle By Name(cluster=w37, "Update Display"=FALSE, "Left Motor"=w33, "Right Motor Ref"=w77) -> (w76:T29)
  }
  n133 = flat-sequence {
    frame #0 {
      (unwired) ENUM_CMD_Mode_Select."STOP"  # ACT Input.Mode
      (unwired) ENUM_ACT_Action."Open HW Only" ("Action")
      (unwired) ENUM_ACT_State."Startup" ("State")
      (unwired) ENUM_ACT_Action."Config HW Get" ("Action")
      # "State LIST"
      # "Action LIST"
    }
  }
  n134 = Unbundle By Name(w23) -> ("Right Motor Ref"=w17:T21, "Left Motor"=w4:T21)
  n135 = flat-sequence {
    tunnel: w17 -> [w415]
    tunnel: w4 -> [w412]
    frame #0 {
      n136 = call <vilib>:"WPI_MotorControlDisable.vi"("MotorControlDevRef"=w415) -> ("error out"=w413:errorcluster)  [unwired: 9 in, 1 out]
      n137 = local write "CMD Override"(T2."Teleop-Auto" ("CMD Override")) -> ()
      n138 = call <vilib>:"WPI_MotorControlDisable.vi"("error in (no error)"=w413, "MotorControlDevRef"=w412) -> ()  [unwired: 8 in, 2 out]
    }
  }
